vi "Configure Current Limit.vi"(6 "Trigger Source (0: Immediate)":i32(ring) items=["Immediate", "Triggered"], 8 "error in (no error)":errorcluster, 9 "Current Limit (0.0 A)":dbl min=0.0 max=420.0 format="%.2g", 10 "Enable Current Protection (F: Disable)":bool, 11 "VISA resource name":refnum<visa-resource-name>) -> (0 "error out":errorcluster, 3 "VISA resource name out":refnum<visa-resource-name>)   [LabVIEW 2014, in "Agilent N87XX Series.lvlib"]
doc: "Configures over current protection (OCP). Specify the output current limit value and the behavior of the power supply when the output current is greater than or equal to that value. If you set the limit for the triggered state, you can send a trigger with the Send Software Trigger VI."
uses:
  Agilent N87XX Series.lvlib
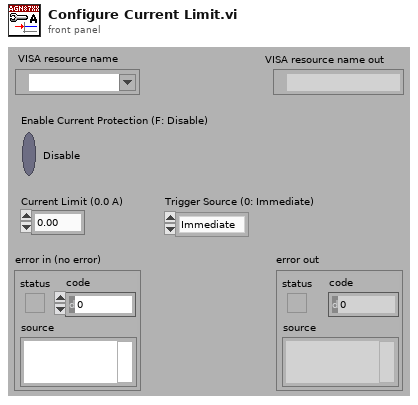
[diagram p1: front panel]
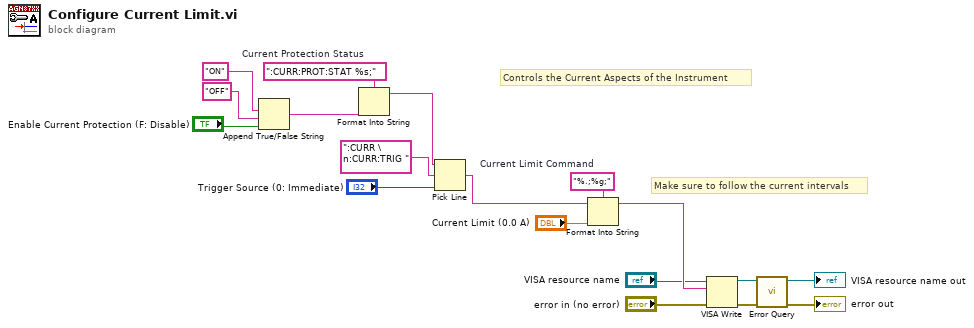
[diagram p0: block diagram]
diagram:
  w9 = ":CURR:PROT:STAT %s;"  # Current Protection Status
  w10 = "%.;%g;"  # Current Limit Command
  # "Make sure to follow the current intervals"
  # "Controls the Current Aspects of the Instrument"
  n1 = Append True/False String(1:"Enable Current Protection (F: Disable)", 2:"OFF", 3:"ON") -> (0:w5:string)  [unwired: 1 in]
  n2 = Format Into String(format string=w9, w5) -> (resulting string=w2:string)  [unwired: 2 in, 1 out]
  n3 = Pick Line(string ("")=w2, multi-line string=":CURR \n:CURR:TRIG ", line index="Trigger Source (0: Immediate)") -> (output string=w1:string)
  n4 = Format Into String(format string=w10, initial string=w1, "Current Limit (0.0 A)") -> (resulting string=w14:string)  [unwired: 1 in, 1 out]
  n5 = VISA Write(VISA resource name="VISA resource name", write buffer=w14, error in (no error)="error in (no error)") -> (VISA resource name out=w16:refnum<visa-resource-name>, error out=w15:errorcluster)  [unwired: 1 out]
  n6 = call "Error Query.vi"("error in (no error)"=w15, "VISA resource name"=w16) -> ("error out"=→"error out":errorcluster, "VISA resource name out"=→"VISA resource name out":refnum<visa-resource-name>)  [unwired: 6 in, 2 out]
